vi "Write Value.vi"(9 "Variant":variant, 10 "Row":i32, 11 "Series in":refnum<class "Series.lvclass">) -> (3 "Series out":refnum<class "Series.lvclass">)   [LabVIEW 2018, in "InfluxDB Client.lvlib" / "Series.lvclass"]
uses:
  Series.lvclass
  <userlib>/_OpenG.lib/dictionary/dictionary.llb/Dictionary Key Value Pair Cluster__ogtk.ctl
  Series.lvclass/Series.ctl
  <userlib>/_OpenG.lib/dictionary/dictionary.llb/Dictionary Update (by scalar value)__ogtk.vi
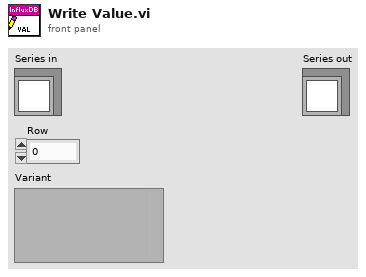
[diagram p1: front panel]
types:
  T1 = typedef "Dictionary Key Value Pair Cluster__ogtk.ctl" = cluster{"key":variant, "value":variant}
  T2 = typedef "Dictionary Object RefNum__ogtk.ctl" = refnum<k1>
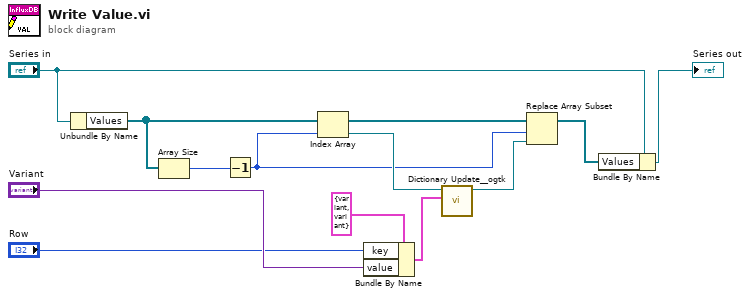
[diagram p0: block diagram]
diagram:
  n1 = Unbundle By Name("Series in") -> ("Values"=w5:T2[])
  n2 = Array Size(array=w5) -> (size(s)=w10:i32)
  n3 = Decrement(x=w10) -> (x-1=w4:i32)
  n4 = Index Array(array=w5, index=w4) -> (element=w9:T2)
  n5 = Bundle By Name(cluster=T1 {"key"=variant, "value"=variant} ("key-value"), "key"="Row", "value"="Variant") -> (w6:T1)
  n6 = call-poly <userlib>:"Dictionary Update__ogtk.vi"("key-value"=w6, "dictionary"=w9) -> ("dictionary out"=w3:T2)  [unwired: 7 in, 2 out]
  n7 = Replace Array Subset(array=w5, new element=w3, index=w4) -> (w2:T2[])
  n8 = Bundle By Name(cluster="Series in", "Values"=w2) -> (→"Series out":refnum<class "Series.lvclass">)
